vi "rspvtd_Get Data.vi"(8 "error in":errorcluster, 11 "Data in":variant) -> (0 "error out":errorcluster, 3 "Data out":T1=variant(string ""))   [LabVIEW 2023, in "Abstract Hardware.lvlib" / "Base Hardware.lvclass"]
doc: "This VI converts variant data contained in the associated <b>Public API Response</b> message to its correct data type.\n---"
uses:
  Base Hardware.lvclass
  rsp_Get Data.ctl
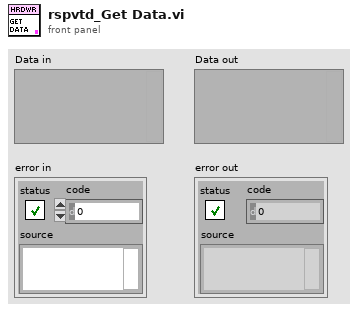
[diagram p1: front panel]
types:
  T1 = typedef "Abstract Hardware.lvlib/Base Hardware.lvclass/rsp_Get Data.ctl" = variant
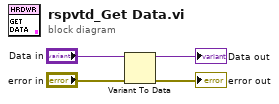
[diagram p0: block diagram]
diagram:
  n1 = Variant To Data(error in="error in", Variant="Data in") -> (data=→"Data out":T1, error out=→"error out":errorcluster)  [unwired: 1 in]
